vi "Discover Unique Names of Dependencies.vi"(0 "NIPKG_LV in":refnum<class "NIPKG_LV.lvclass">) -> (4 "NIPKG_LV out":refnum<class "NIPKG_LV.lvclass">)   [LabVIEW 2017, in "CL_G3_VIComponentBuilder.lvlib" / "NIPKG_LV.lvclass"]
doc: "Interrogates this exports dependencies for thier unique names (as opposed to the product name of the dependency). The unique names are used when assembling the working set of exports in order to prevent name collisions and allow the build analyzer to determine the build order."
uses:
  NIPKG_LV.lvclass
  C:/Tool Chain Support/Software Module Builder/Source/Exports/Exports/Export.lvclass
  Exports/Export.lvclass/Export.ctl
  Exports/Accessors/Read Export Build Specification.vi
  Exports/Accessors/Read Export Operation Errors.vi
  <vilib>/xml/Close Reference(Node).vi
  Exports/Accessors/Write Dependencies' Unique Names.vi
  NI Build Specification_LV/NI Build Specification_LV.lvclass
  <vilib>/xml/NI_XML.lvlib
  <resource>/objmgr/DOMUserDefRef.rc
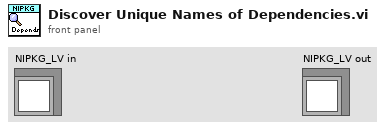
[diagram p1: front panel]
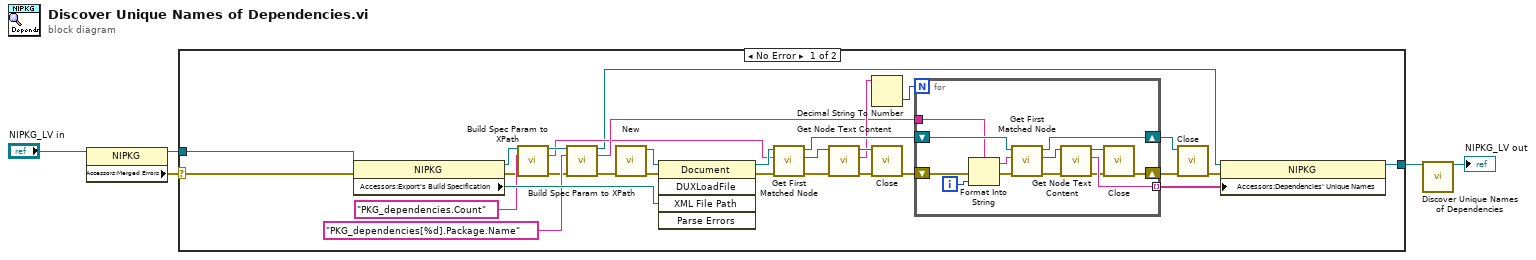
[diagram p0: block diagram]
diagram:
  n1 = property class="NIPKG"(reference="NIPKG_LV in") -> (reference out=w4:refnum<class "NIPKG_LV.lvclass">, "Accessors:Merged Errors"=w1:errorcluster)  [unwired: 1 in, 1 out]
  n2 = case shown="No Error" w1 {
    selector: w1 -> [w18 _]
    tunnel: w4 -> [w35 w49]
    tunnel: [w33 w49] -> w3
    frame No Error {
      n3 = property class="NIPKG"(reference=w35, error in=w18) -> (reference out=w16:refnum<class "NIPKG_LV.lvclass">, error out=w8:errorcluster, "Accessors:Export's Build Specification"=w17:path)
      n4 = call-dynamic "Build Spec Param to XPath.vi"("NI Build Specification"=w16, "Build Spec Parameter Name"="PKG_dependencies.Count", "error in (no error)"=w8) -> ("NI Build Specification"=w15:refnum<class "NIPKG_LV.lvclass">, "XPath to the specific build Spec Property"=w11:string, "error out"=w7:errorcluster)  [unwired: 10 in]
      n5 = call-dynamic "Build Spec Param to XPath.vi"("NI Build Specification"=w15, "Build Spec Parameter Name"="PKG_dependencies[%d].Package.Name", "error in (no error)"=w7) -> ("NI Build Specification"=w9:refnum<class "NIPKG_LV.lvclass">, "XPath to the specific build Spec Property"=w12:string, "error out"=w6:errorcluster)  [unwired: 10 in]
      n6 = call <vilib>:"New.vi"("error in (no error)"=w6) -> ("error out"=w19:errorcluster, "DOM document out"=w20:refnum<k20>)  [unwired: 7 in]
      n7 = invoke class="Document" method="DUXLoadFile"(reference=w20, error in=w19, "XML File Path"=w17) -> (reference out=w23:refnum<k20>, error out=w10:errorcluster)  [unwired: 2 in, 3 out]
      n8 = call <vilib>:"Get First Matched Node.vi"("error in (no error)"=w10, "XPath expression"=w11, "node in"=w23) -> ("error out"=w22:errorcluster, "node result"=w21:refnum<k20>, "node out"=w25:refnum<k20>)  [unwired: 6 in]
      n9 = call <vilib>:"Get Node Text Content.vi"("error in (no error)"=w22, "node in"=w21) -> ("error out"=w29:errorcluster, "node text"=w24:string, "node out"=w31:refnum<k20>)  [unwired: 7 in]
      n10 = Decimal String To Number(string=w24) -> (number=w28:i32)  [unwired: 2 in, 1 out]
      n11 = call-poly <vilib>:"Close.vi"("error in (no error)"=w29, "node"=w31) -> ("error out"=w30:errorcluster)  [unwired: 7 in]
      n12 = for {
        N: w28 -> [_]
        shift-right: [w41] -> w27
        shift-left: w25 -> [w48]
        shift-right: [w38] -> w26
        shift-left: w30 -> [w43]
        tunnel: w12 -> [w47]
        tunnel: [w42] -> w34 mode=indexing
        i -> [w36]
        n13 = Format Into String(format string=w47, error in=w43, w36) -> (resulting string=w46:string, error out=w40:errorcluster)  [unwired: 1 in]
        n14 = call <vilib>:"Get First Matched Node.vi"("error in (no error)"=w40, "XPath expression"=w46, "node in"=w48) -> ("error out"=w45:errorcluster, "node result"=w44:refnum<k20>, "node out"=w41:refnum<k20>)  [unwired: 6 in]
        n15 = call <vilib>:"Get Node Text Content.vi"("error in (no error)"=w45, "node in"=w44) -> ("error out"=w39:errorcluster, "node text"=w42:string, "node out"=w37:refnum<k20>)  [unwired: 7 in]
        n16 = call-poly <vilib>:"Close.vi"("error in (no error)"=w39, "node"=w37) -> ("error out"=w38:errorcluster)  [unwired: 7 in]
      }
      n17 = call-poly <vilib>:"Close.vi"("error in (no error)"=w26, "node"=w27) -> ("error out"=w32:errorcluster)  [unwired: 7 in]
      n18 = property class="NIPKG"(reference=w9, error in=w32, "Accessors:Dependencies' Unique Names"=w34) -> (reference out=w33:refnum<class "NIPKG_LV.lvclass">)  [unwired: 1 out]
    }
    frame Error {
    }
  }
  n19 = call-parent "Discover Unique Names of Dependencies.vi"("NI Build Specification_LV In"=w3) -> ("NI Build Specification_LV Out"=→"NIPKG_LV out":refnum<class "NIPKG_LV.lvclass">)  [unwired: 14 in]
